vi "Read difftrack.vi"(8 "error in (no error)":errorcluster, 11 "Target in":refnum<class "Target.lvclass">) -> (0 "error out":errorcluster, 2 "Difftrack.lvclass":refnum<class "Difftrack.lvclass">, 3 "Target out":refnum<class "Target.lvclass">)   [LabVIEW 2022 SP3, in "TCSDataDefinitions.lvlib" / "TCSCommand.lvlib" / "TargetConfiguration.lvlib" / "Target.lvlib" / "Target.lvclass"]
uses:
  Target/Target.lvclass
  Difftrack/Difftrack.lvclass
  Target/Target.lvclass/Target.ctl
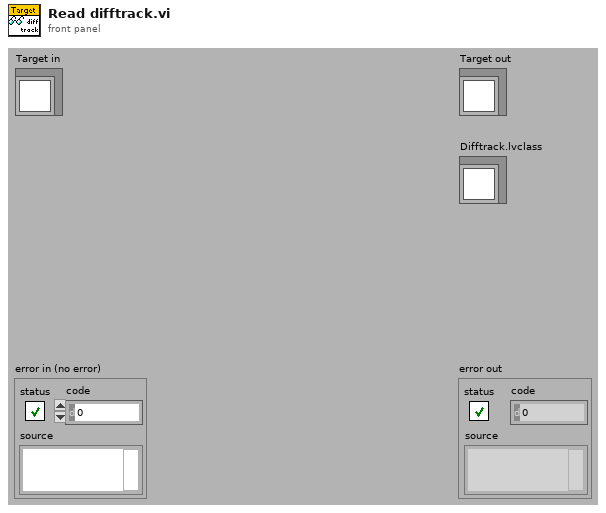
[diagram p1: front panel]
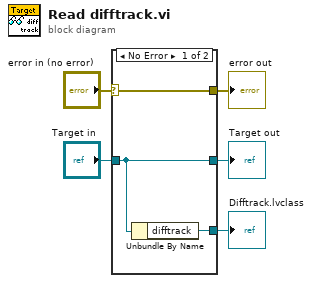
[diagram p0: block diagram]
diagram:
  n1 = case shown="No Error" "error in (no error)" {
    selector: "error in (no error)" -> [w8 w9]
    tunnel: [w8 w9] -> w4
    tunnel: [w7 w10] -> w2
    tunnel: "Target in" -> [w7 w10]
    tunnel: [w6 _] -> w1
    frame No Error {
      n2 = Unbundle By Name(w7) -> ("difftrack"=w6:refnum<class "Difftrack.lvclass">)
    }
    frame Error {
    }
  }
  "error out" <- w4
  "Target out" <- w2
  "Difftrack.lvclass" <- w1
